vi "vi.highlight-control-by-index.vi"(8 "error in (no error)":errorcluster, 10 "control index":i32, 11 "selected VI":path) -> (0 "error out":errorcluster)   [LabVIEW 2020]
uses:
  <vilib>/ErrorRing/Error Ring.xnode
  <vilib>/Utility/error.llb/Error Cluster From Error Code.vi
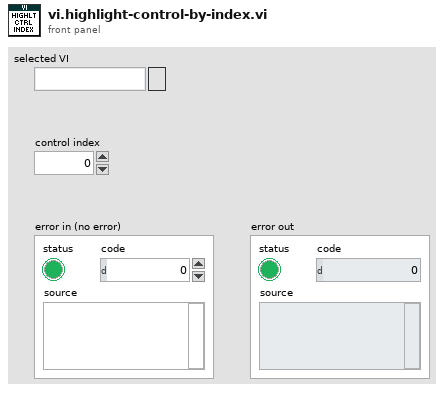
[diagram p1: front panel]
types:
  T1 = enum32{"Invalid", "Standard", "Closed", "Hidden", "Minimized", "Maximized"}
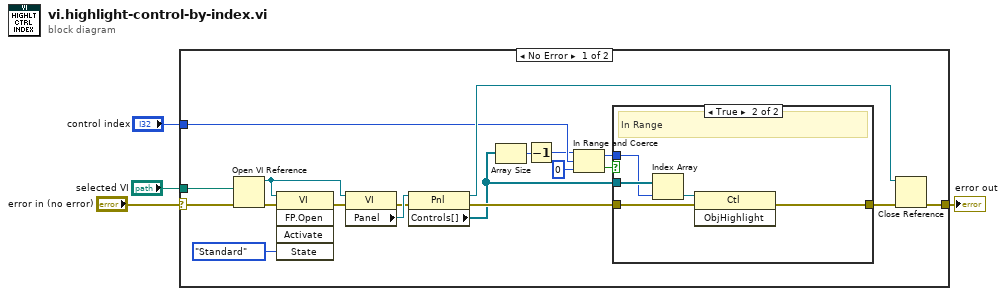
[diagram p0: block diagram]
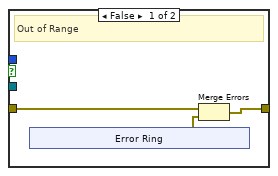
[diagram p2: hidden frame]
diagram:
  n1 = case shown="No Error" "error in (no error)" {
    selector: "error in (no error)" -> [w16 w37]
    tunnel: [w19 w37] -> w4
    tunnel: "selected VI" -> [w13 _]
    tunnel: "control index" -> [w12 _]
    frame No Error {
      n2 = Open VI Reference(vi path=w13, error in (no error)=w16) -> (vi reference=w21:refnum<vi>, error out=w5:errorcluster)  [unwired: 4 in]
      n3 = invoke class="VI" method="FP.Open"(reference=w21, error in=w5, "State"=T1."Standard") -> (error out=w23:errorcluster)  [unwired: 2 in, 4 out]
      n4 = property class="VI"(reference=w21, error in=w23) -> (error out=w14:errorcluster, "Panel"=w20:refnum<vi>)  [unwired: 1 out]
      n5 = property class="Pnl"(reference=w20, error in=w14) -> (reference out=w15:refnum<vi>, error out=w17:errorcluster, "Controls[]"=w10:refnum<vi>[])
      n6 = Array Size(array=w10) -> (size(s)=w9:i32)
      n7 = Decrement(x=w9) -> (x-1=w8:i32)
      n8 = In Range and Coerce(upper limit=w8, x=w12, lower limit=0) -> (coerced(x)=w7:i32, In Range?=w6:bool)
      n9 = case shown="True" w6 {
        tunnel: [w25 w36] -> w18
        tunnel: w17 -> [w26 w35]
        tunnel: w10 -> [_ w33]
        tunnel: w7 -> [_ w32]
        frame False {
          # "Out of Range"
          n10 = xnode "Error Ring"() -> ("error out"=w24:errorcluster)
          n11 = Merge Errors(w26, w24) -> (w25:errorcluster)
        }
        frame True {
          # "In Range"
          n12 = Index Array(array=w33, index=w32) -> (element=w34:refnum<vi>)
          n13 = invoke class="Ctl" method="ObjHighlight"(reference=w34, error in=w35) -> (error out=w36:errorcluster)  [unwired: 1 in, 2 out]
        }
      }
      n14 = Close Reference(reference=w15, error in (no error)=w18) -> (error out=w19:errorcluster)
    }
    frame Error {
    }
  }
  "error out" <- w4
